vi "receiver.vi"() -> ()   [LabVIEW 2013]
uses:
  <instrlib>/niUSRP/niUSRP Fetch Rx Data (CDB WDT).vi
  <vilib>/express/express analysis/Spectral/Block/exnSpectralBlock spectral measurements RMS poly.vi
  <vilib>/express/express analysis/Spectral/Block/exnSpectralBlock spectral measurements RMS WFM.vi
  <vilib>/express/express analysis/Spectral/XNode/ExpressSpectralMeasurementsBlockNode.xnode
panel:
  in  "number of samples":i64=1000
  in  "active antenna":string
  in  "gain":dbl
  in  "carrier frequency":dbl
  in  "IQ rate":dbl
  in  "stop":bool
  in  "device names":refnum<k15>
  out "coerced gain":dbl format="%#_6f"
  out "coerced carrier frequency":dbl=100000.0 format="%#_6p"
  out "coerced IQ rate":dbl=100000.0 format="%#_6p"
  out "Spectrum":cluster{"f0":dbl, "df":dbl, "magnitude":dbl[]}(graph)
  out "Waveform Graph":waveform(dbl)[](graph)
  out "error out":errorcluster
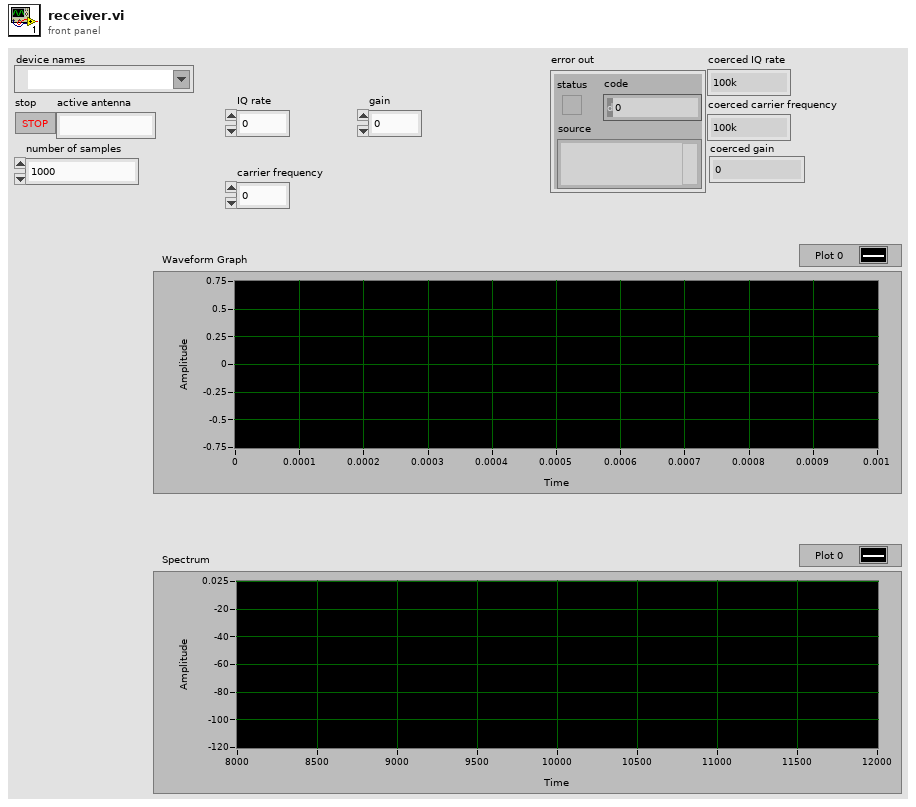
[diagram p1: front panel]
types:
  T1 = cluster{"averaging mode":u16, "weighting mode":u16, "number of averages":u32}
  T2 = cluster{"dB On (F)":bool, "unwrap phase (F)":bool, "convert to degree (F)":bool}
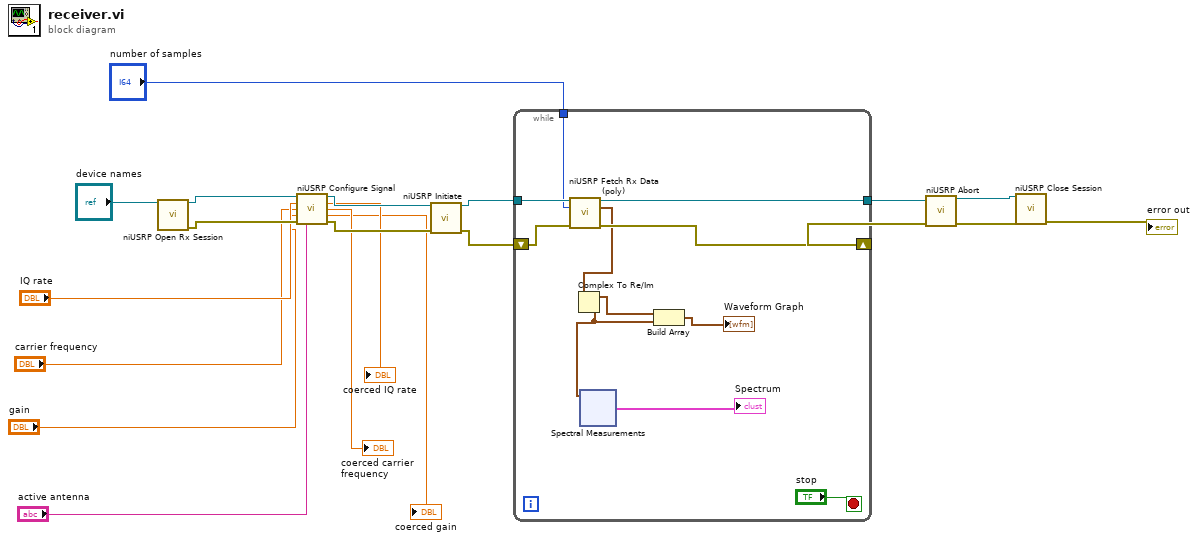
[diagram p0: block diagram]
diagram:
  n1 = call <instrlib>:"niUSRP Open Rx Session.vi"("device names"="device names") -> ("session handle out"=w19:refnum<k15>, "error out"=w14:errorcluster)  [unwired: 13 in]
  n2 = call <instrlib>:"niUSRP Configure Signal.vi"("session handle"=w19, "IQ rate"="IQ rate", "carrier frequency"="carrier frequency", "gain"="gain", "error in (no error)"=w14, "active antenna"="active antenna") -> ("session handle out"=w18:refnum<k15>, "coerced IQ rate"=→"coerced IQ rate":dbl, "coerced carrier frequency"=→"coerced carrier frequency":dbl, "coerced gain"=→"coerced gain":dbl, "error out"=w13:errorcluster)  [unwired: 5 in]
  n3 = call <instrlib>:"niUSRP Initiate.vi"("session handle"=w18, "error in (no error)"=w13) -> ("session handle out"=w17:refnum<k15>, "error out"=w12:errorcluster)  [unwired: 12 in]
  n4 = while {
    tunnel: w17 -> [w31]
    tunnel: [w30] -> w16
    shift-right: [w28] -> w11
    shift-left: w12 -> [w29]
    tunnel: "number of samples" -> [w22]
    stop <- "stop" stop-if-true
    n5 = call-poly <instrlib>:"niUSRP Fetch Rx Data (poly).vi"("session handle"=w31, "number of samples"=w22, "error in (no error)"=w29) -> ("session handle out"=w30:refnum<k15>, "data"=w27:waveform(cdb), "error out"=w28:errorcluster)  [unwired: 9 in, 1 out]
    n6 = Complex To Re/Im(x + iy=w27) -> (x=w26:waveform(dbl), y=w21:waveform(dbl))
    n7 = xnode "Spectral Measurements"("Signals"=w21) -> ("FFT - (RMS)"=→"Spectrum":cluster{"f0":dbl, "df":dbl, "magnitude":dbl[]})  [unwired: 1 in, 2 out]
    n8 = Build Array(w26, w21) -> (→"Waveform Graph":waveform(dbl)[])
  }
  n9 = call <instrlib>:"niUSRP Abort.vi"("session handle"=w16, "error in (no error)"=w11) -> ("session handle out"=w15:refnum<k15>, "error out"=w10:errorcluster)  [unwired: 12 in]
  n10 = call <instrlib>:"niUSRP Close Session.vi"("session handle"=w15, "error in (no error)"=w10) -> ("error out"=→"error out":errorcluster)  [unwired: 13 in]
